vi "PreCheck.vi"(8 "Error In (No Error)":errorcluster, 10 "Pre-Check Cut-Off (V)":dbl=0.5, 11 "Potentiostat":refnum<visa-resource-name>="Solartron1287") -> (0 "Error Out":errorcluster, 1 "Pre-Check Voltage":dbl(graph), 2 "Characters Read":string, 3 "Potentiostat":refnum<visa-resource-name>="Solartron1287", 4 "<Cut-Off?":bool, 5 "Error code 2":dbl, 6 "No potentiostat Error?":bool, 7 "Error code 1":dbl)   [LabVIEW 2018]
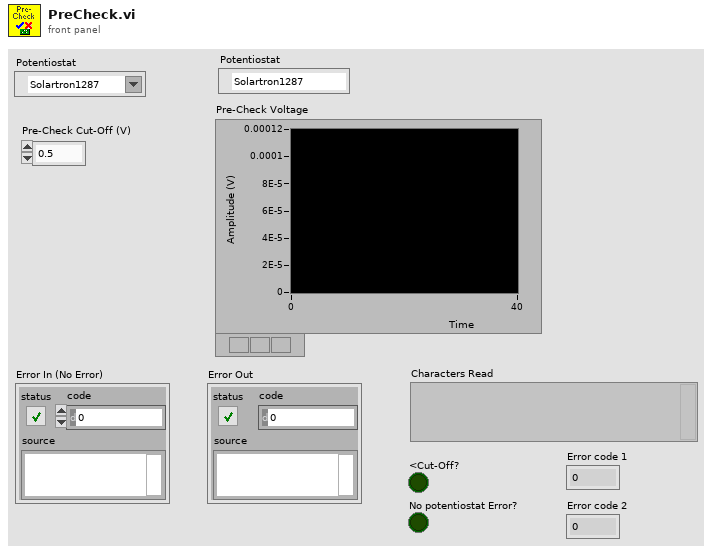
[diagram p1: front panel]
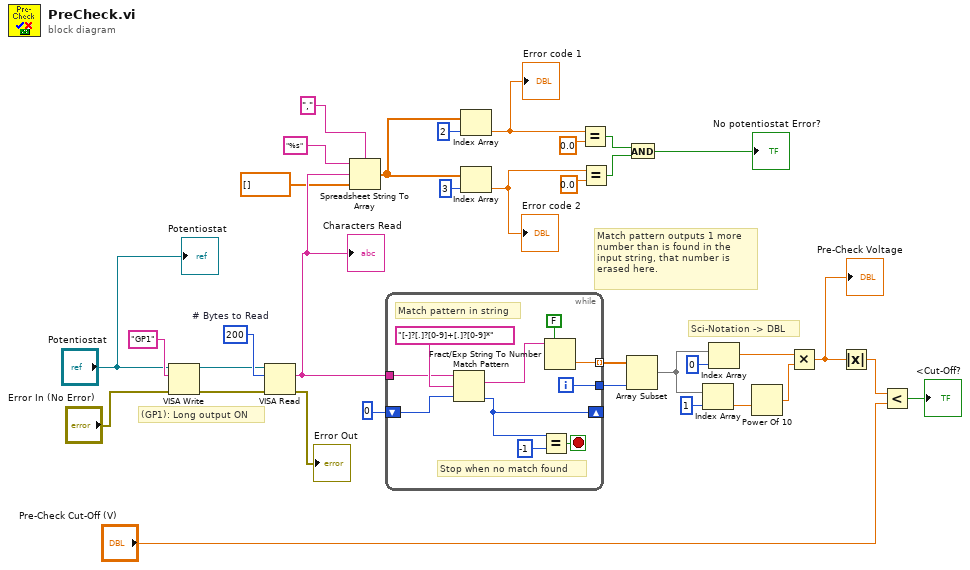
[diagram p0: block diagram]
diagram:
  w22 = 200  # # Bytes to Read
  # "(GP1): Long output ON"
  # "Sci-Notation -> DBL"
  # "Match pattern outputs 1 more\nnumber than is found in the \ninput string, that number is\nerased here."
  n1 = VISA Write(VISA resource name="Potentiostat", write buffer="GP1" ("Characters to Write"), error in (no error)="Error In (No Error)") -> (VISA resource name out=w20:refnum<visa-resource-name>, error out=w21:errorcluster)  [unwired: 1 out]
  n2 = VISA Read(VISA resource name=w20, byte count=w22, error in (no error)=w21) -> (read buffer=w14:string, error out=→"Error Out":errorcluster)  [unwired: 2 out]
  "Characters Read" <- w14
  n3 = Spreadsheet String To Array(delimiter (Tab)=",", format string="%s", spreadsheet string=w14, array type (2D Dbl)=dbl[] []) -> (array=w8:dbl[])
  n4 = while {
    tunnel: w14 -> [w42]
    tunnel: [w44] -> w33
    shift-left: 0 -> [w38]
    shift-right: [w37] -> _
    tunnel: [w41] -> w32 mode=indexing
    i -> [w44]
    stop <- w40 stop-if-true
    # "Stop when no match found"
    # "Match pattern in string"
    n5 = Match Pattern(string=w42, regular expression="[-]?[.]?[0-9]+[.]?[0-9]*", offset (0)=w38) -> (match substring=w36:string, offset past match=w37:i32)  [unwired: 2 out]
    n6 = Equal?(x=w37, y=-1) -> (x = y?=w40:bool)
    n7 = Fract/Exp String To Number(use system decimal point (T)=FALSE, string=w36) -> (number=w41:dbl)  [unwired: 2 in, 1 out]
  }
  n8 = Index Array(array=w8, index=2) -> (element=w7:dbl)
  "Error code 1" <- w7
  n9 = Index Array(array=w8, index=3) -> (element=w4:dbl)
  "Error code 2" <- w4
  n10 = Equal?(x=w7, y=0.0) -> (x = y?=w3:bool)
  n11 = Equal?(x=w4, y=0.0) -> (x = y?=w2:bool)
  n12 = Array Subset(array=w32, length=w33) -> (w29:dbl[])  [unwired: 1 in]
  n13 = And(x=w3, y=w2) -> (x .and. y?=→"No potentiostat Error?":bool)
  n14 = Index Array(array=w29, index=1) -> (element=w27:dbl)
  n15 = Index Array(array=w29, index=0) -> (element=w28:dbl)
  n16 = Power Of 10(x=w27) -> (10^x=w26:dbl)
  n17 = Multiply(x=w28, y=w26) -> (x*y=w23:dbl)
  "Pre-Check Voltage" <- w23
  n18 = Absolute Value(x=w23) -> (abs(x)=w24:dbl)
  n19 = Less?(x=w24, y="Pre-Check Cut-Off (V)") -> (x < y?=→"<Cut-Off?":bool)
  "Potentiostat" <- "Potentiostat"
